vi "CheckTableIsNumeric.vi"(8 "ErrorArray In":errorcluster[](array[cluster]), 9 "strOldVal":string[][](array[string]), 10 "strNewVal":string[][](array[string]), 11 "TableRefnum":refnum<vi>) -> (0 "ErrorArray Out":errorcluster[](array[cluster]))   [LabVIEW 2017, in "Framework.lvlib"]
uses:
  Framework.lvlib
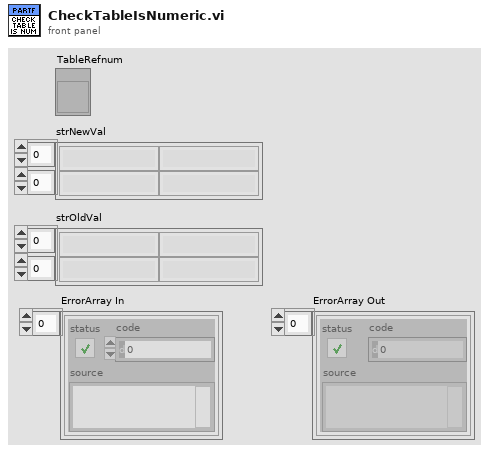
[diagram p1: front panel]
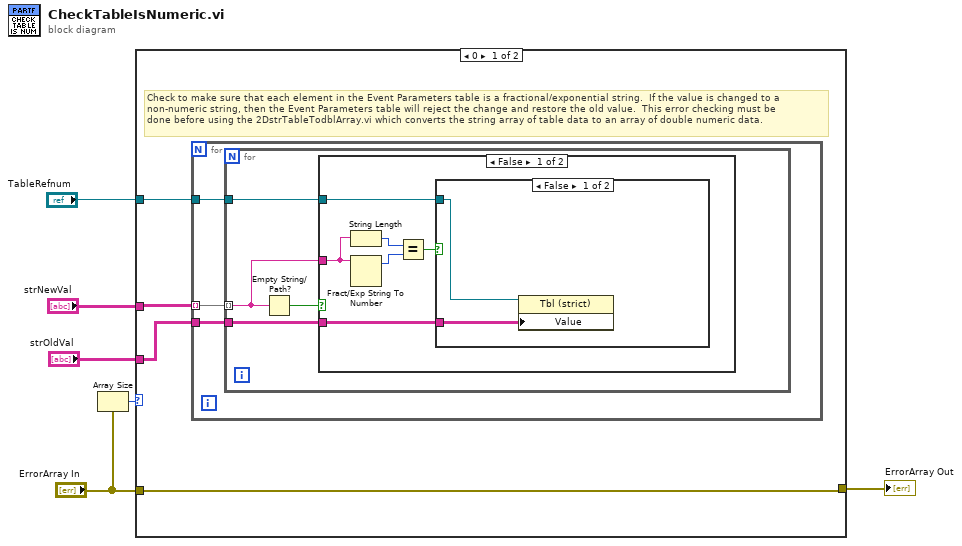
[diagram p0: block diagram]
diagram:
  n1 = Array Size(array="ErrorArray In") -> (size(s)=w5:i32)
  n2 = case shown="0" w5 {
    tunnel: "ErrorArray In" -> [w7 w26]
    tunnel: [w7 w26] -> w6
    tunnel: "strOldVal" -> [w9 _]
    tunnel: "strNewVal" -> [w10 _]
    tunnel: "TableRefnum" -> [w8 _]
    frame 0 {
      # "Check to make sure that each element in the Event Parameters table is a fractional/exponential string.  If the value is changed to a\nnon-numeric string, then the Event Parameters table will reject the change and restore the old value.  This error checking must be\ndone before using the 2DstrTableTodblArray.vi which converts the string array of table data to an array of double numeric data."
      n3 = for {
        tunnel: w10 -> [w13] mode=indexing
        tunnel: w9 -> [w12]
        tunnel: w8 -> [w11]
        n4 = for {
          tunnel: w13 -> [w16] mode=indexing
          tunnel: w12 -> [w15]
          tunnel: w11 -> [w14]
          n5 = Empty String/Path?(string/path=w16) -> (empty?=w17:bool)
          n6 = case shown="False" w17 {
            tunnel: w16 -> [w23 _]
            tunnel: w15 -> [w19 _]
            tunnel: w14 -> [w18 _]
            frame False {
              n7 = String Length(string=w23) -> (length=w21:i32)
              n8 = Fract/Exp String To Number(string=w23) -> (offset past number=w22:i32)  [unwired: 3 in, 1 out]
              n9 = Equal?(x=w21, y=w22) -> (x = y?=w20:bool)
              n10 = case shown="False" w20 {
                tunnel: w19 -> [w25 _]
                tunnel: w18 -> [w24 _]
                frame False {
                  n11 = property on="Property Node" class="Tbl (strict)"(reference=w24, "Value"=w25) -> ()  [unwired: 1 in, 2 out]
                }
                frame True {
                }
              }
            }
            frame True {
            }
          }
        }
      }
    }
    frame 1, Default {
    }
  }
  "ErrorArray Out" <- w6
